vi "Reboot_Trimming_Registers.vi"(7 "I2C Channel":u8, 8 "error in (no error)":errorcluster, 11 "LINX Resource In":T1) -> (0 "error out":errorcluster, 3 "LINX Resource Out":T1)   [LabVIEW 2014, in "LMH-LINX.lvlib" / "LIS331HH.lvlib"]
doc: "BOOT bit is used to refresh the content of internal registers stored in the flash memory block.\nAt the end of the boot process the BOOT bit CTRL_REG2[8]is set again to ‘0’s\n\n**Author: Stas Legedza"
uses:
  <vilib>/MakerHub/LINX/Public/Sensors/Accelerometer/LIS331HH/LIS331HH.lvlib
  <vilib>/MakerHub/LINX/Private/Type Defs/LINX Ref.ctl
  <vilib>/MakerHub/LINX/Private/Type Defs/Platform.ctl
  <vilib>/MakerHub/LINX/Private/Type Defs/Interface.ctl
  <vilib>/MakerHub/LINX/Private/Device/Type Defs/LINX Device Config.ctl
  <vilib>/MakerHub/LINX/Private/Device/Type Defs/TCP Config.ctl
  <vilib>/MakerHub/LINX/Private/Device/Type Defs/Channels.ctl
  <vilib>/MakerHub/LINX/Private/Local IO/LinxI2cWrite.vi
  <vilib>/MakerHub/LINX/Public/Utilities/Check Channel.vi
  <vilib>/MakerHub/LINX/Private/Utilties/Generate Error.vi
  <vilib>/MakerHub/LINX/LMH-LINX.lvlib
  <vilib>/MakerHub/LINX/Private/Device/Device.lvlib
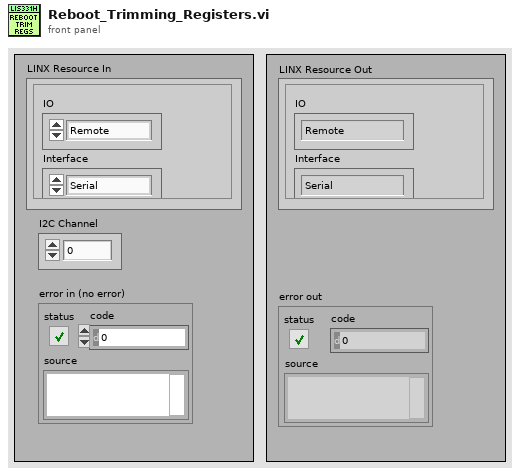
[diagram p1: front panel]
types:
  T1 = typedef "LMH-LINX.lvlib/LINX Ref.ctl" = cluster{"IO":T2, "Interface":T3, "LINX Device Config":T4}
  T2 = typedef "LMH-LINX.lvlib/Platform.ctl" = enum16{"Remote", "Local"}
  T3 = typedef "LMH-LINX.lvlib/Interface.ctl" = enum16{"Serial", "TCP"}
  T4 = typedef "LMH-LINX.lvlib/Device.lvlib/LINX Device Config.ctl" = cluster{"Interface":T3, "COM Port":refnum<visa-resource-name>, "TCP Configuration":T5, "Device Family":u8, "Device ID":u8, "Device Name":string, "TCP Ref":refnum<k5>, "Channels":T6}
  T5 = typedef "LMH-LINX.lvlib/Device.lvlib/TCP Config.ctl" = cluster{"IP Address":string, "Port":u16}
  T6 = typedef "LMH-LINX.lvlib/Channels.ctl" = cluster{"DI":u8[], "DO":u8[], "AI":u8[], "AO":u8[], "PWM":u8[], "QE":u8[], "UART":u8[], "I2C 2":u8[], "SPI":u8[], "CAN":u8[], "Servo":u8[], "AI Ref (V)":dbl, "AI Resolution (Bits)":u8, "AO Ref (V)":dbl, "AO Resolution (Bits)":u8}
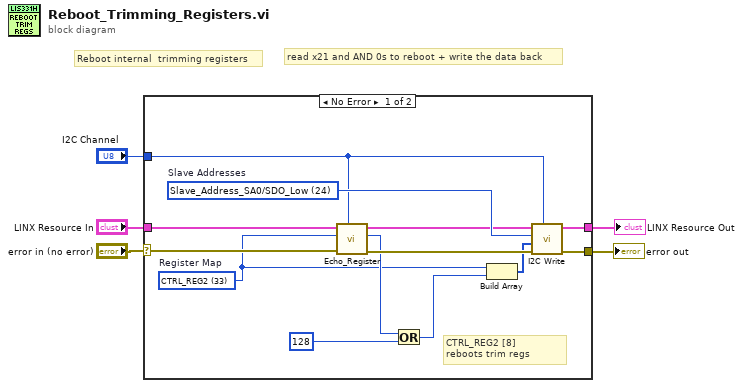
[diagram p0: block diagram]
diagram:
  # "read x21 and AND 0s to reboot + write the data back"
  # "Reboot internal  trimming registers"
  n1 = case shown="No Error" "error in (no error)" {
    selector: "error in (no error)" -> [w14 w20]
    tunnel: [w17 w20] -> w4
    tunnel: "LINX Resource In" -> [w15 w19]
    tunnel: "I2C Channel" -> [w13 _]
    tunnel: [w16 w19] -> w1
    frame No Error {
      w6 = u8 33 items=["CTRL_REG1"=32, "CTRL_REG2"=33, "CTRL_REG3"=34, "CTRL_REG4"=35, "CTRL_REG5"=36, "HP_FILTER_RESET"=37, "REFERENCE"=38, "STATUS_REG"=39, "OUT_X_L"=40, "OUT_X_H"=41, "OUT_Y_L"=42, "OUT_Y_H"=43, "OUT_Z_L"=44, "OUT_Z_H"=45, "INT1_CFG"=48, "INT1_SOURCE"=49, "INT1_THS"=50, "INT1_DURATION"=51, "INT2_CFG"=52, "INT2_SOURCE"=53, "INT2_THS"=54, "INT2_DURATION"=55]  # Register Map
      w18 = u8 24 items=["Slave_Address_SA0/SDO_Low"=24, "Slave_Address_SA0/SDO_High"=25]  # Slave Addresses
      # "CTRL_REG2 [8]\nreboots trim regs"
      n2 = call <vilib>:"Echo_Register.vi"("I2C Channel"=w13, "error in (no error)"=w14, "Register to Echo"=w6, "LINX Resource In"=w15) -> ("error out"=w11:errorcluster, "Register Word"=w9:u8, "LINX Resource Out"=w12:T1)  [unwired: 5 in]
      n3 = Or(x=w9, y=u8 128) -> (x .or. y?=w7:u8)
      n4 = Build Array(w6, w7) -> (w8:u8[])
      n5 = call <vilib>:"I2C Write.vi"("I2C Channel"=w13, "Error In"=w11, "Data"=w8, "I2C Slave Address (0)"=w18, "LINX Resource"=w12) -> ("Error Out"=w17:errorcluster, "LINX Resource"=w16:T1)  [unwired: 5 in]
    }
    frame Error {
    }
  }
  "error out" <- w4
  "LINX Resource Out" <- w1
